vi "test - Enum.vi"(8 "error in (no error)":errorcluster, 11 "TestCase in":refnum<class "testcase-Supported-Datatype.lvclass">) -> (0 "error out":errorcluster, 3 "TestCase out":refnum<class "testcase-Supported-Datatype.lvclass">)   [LabVIEW 2017, in "testcase-Supported-Datatype.lvclass"]
uses:
  testcase-Supported-Datatype.lvclass
  <vilib>/addons/_JKI Toolkits/VI Tester/TestCase.llb/TestCase.lvclass
  addons/API-String-Arugments-Support/API String Arguments Support.lvlib
  C:/Program Files (x86)/National Instruments/LabVIEW 2017/vi.lib/addons/_JKI Toolkits/VI Tester/TestCase.llb/TestCase.lvclass
panel:
  out "data 3":enum16{"1 - aaaa", "2 - bbbb", "555 - ccccc"}(ring)
  out "data 2":enum16{"1 - aaaa", "2 - bbbb", "555 - ccccc"}(ring)
  out "data":enum16{"aaaa", "bbbb", "ccccc"}(ring)
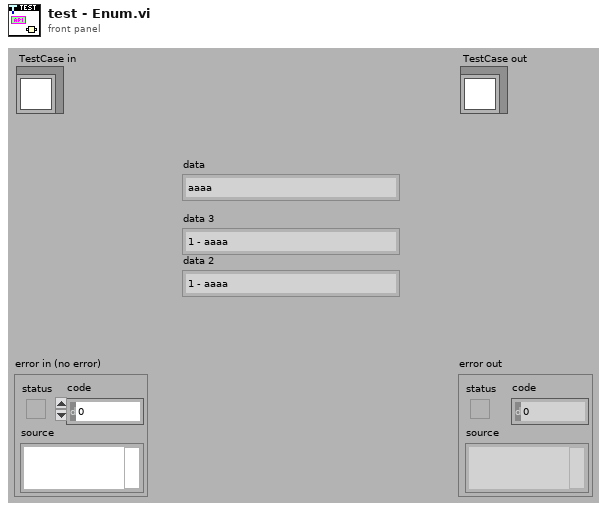
[diagram p1: front panel]
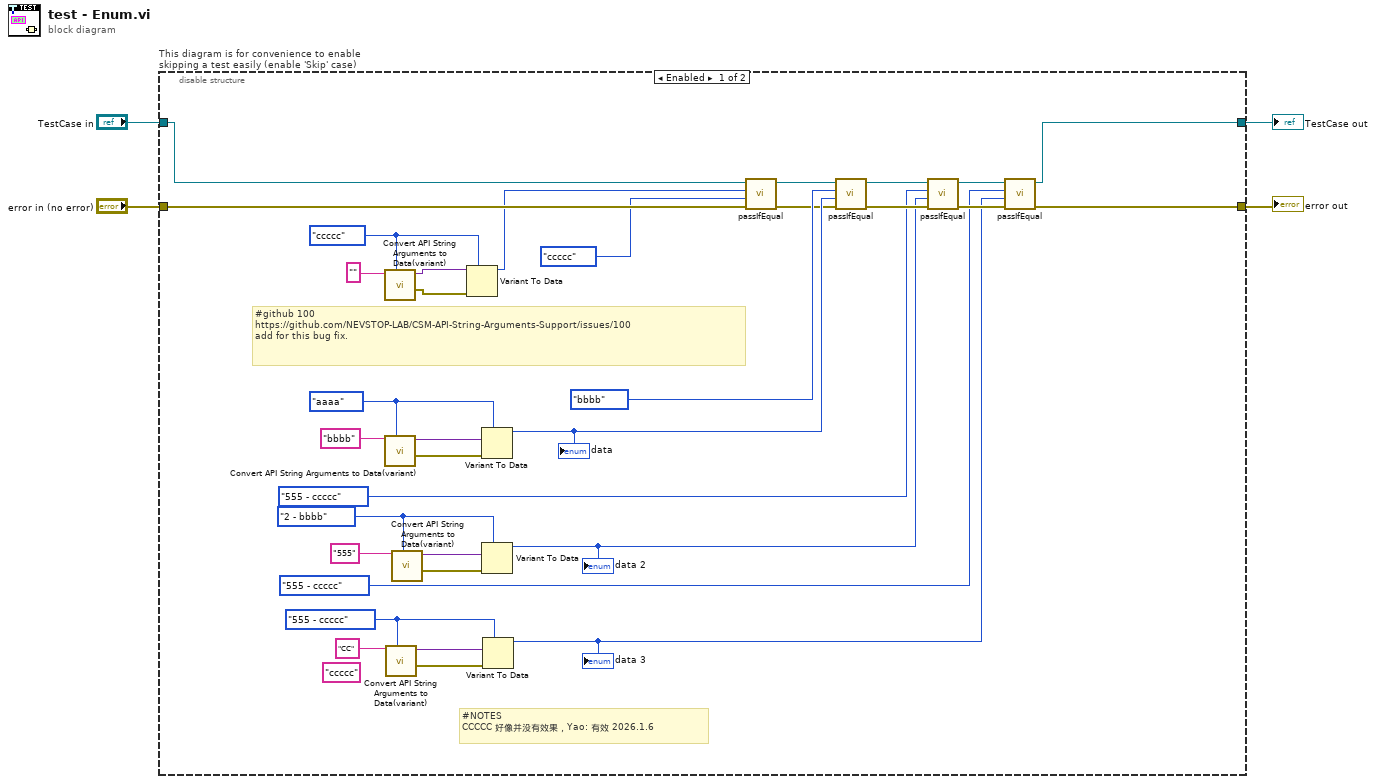
[diagram p0: block diagram]
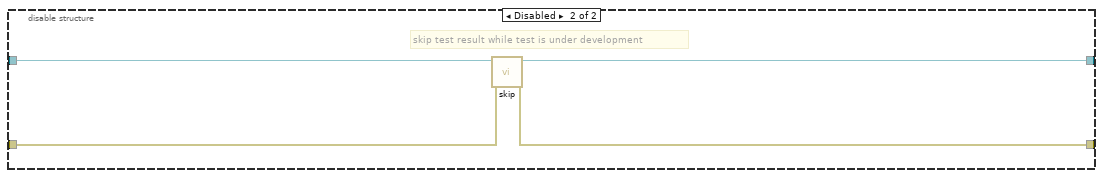
[diagram p2: hidden frame]
diagram:
  n1 = disable-structure "This diagram is for convenience to enable skipping a test easily (enable 'Skip' case)" shown="Enabled" {
    disable-tunnel: "TestCase in" -> [w14 w42]
    disable-tunnel: [w18 w40] -> w1
    disable-tunnel: [w17 w41] -> w3
    disable-tunnel: "error in (no error)" -> [w13 w39]
    frame Enabled {
      (unwired) "ccccc" ("String")
      w7 = enum16{"aaaa", "bbbb", "ccccc"}."ccccc" ("Data 5")
      w21 = enum16{"1 - aaaa", "2 - bbbb", "555 - ccccc"}."555 - ccccc" ("Data 6")
      w29 = enum16{"1 - aaaa", "2 - bbbb", "555 - ccccc"}."2 - bbbb" ("Data 6")
      w35 = enum16{"aaaa", "bbbb", "ccccc"}."aaaa" ("Data 5")
      # "#github 100\nhttps://github.com/NEVSTOP-LAB/CSM-API-String-Arguments-Support/issues/100\nadd for this bug fix."
      # "#NOTES\nCCCCC 好像并没有效果，Yao: 有效 2026.1.6"
      n2 = call "Convert API String Arguments to Data(variant).vi"("Type"=w7, "String"="") -> ("error"=w8:errorcluster, "Data"=w9:variant)  [unwired: 8 in]
      n3 = call "Convert API String Arguments to Data(variant).vi"("Type"=w35, "String"="bbbb") -> ("error"=w38:errorcluster, "Data"=w37:variant)  [unwired: 8 in]
      n4 = call "Convert API String Arguments to Data(variant).vi"("Type"=w21, "String"="CC") -> ("error"=w22:errorcluster, "Data"=w23:variant)  [unwired: 8 in]
      n5 = call "Convert API String Arguments to Data(variant).vi"("Type"=w29, "String"="555") -> ("error"=w30:errorcluster, "Data"=w31:variant)  [unwired: 8 in]
      n6 = Variant To Data(error in=w8, type=w7, Variant=w9) -> (data=w6:enum16{"aaaa", "bbbb", "ccccc"})  [unwired: 1 out]
      n7 = Variant To Data(error in=w38, type=w35, Variant=w37) -> (data=w33:enum16{"aaaa", "bbbb", "ccccc"})  [unwired: 1 out]
      "data" <- w33
      n8 = Variant To Data(error in=w30, type=w29, Variant=w31) -> (data=w25:enum16{"1 - aaaa", "2 - bbbb", "555 - ccccc"})  [unwired: 1 out]
      "data 2" <- w25
      n9 = Variant To Data(error in=w22, type=w21, Variant=w23) -> (data=w15:enum16{"1 - aaaa", "2 - bbbb", "555 - ccccc"})  [unwired: 1 out]
      "data 3" <- w15
      n10 = call-dynamic "passIfEqual.vi"("error in (no error)"=w13, "y"=enum16{"aaaa", "bbbb", "ccccc"}."ccccc" ("Data 5"), "x"=w6, "TestCase in"=w14) -> ("error out"=w12:errorcluster, "TestCase out"=w11:refnum<class "testcase-Supported-Datatype.lvclass">)  [unwired: 6 in]
      n11 = call-dynamic "passIfEqual.vi"("error in (no error)"=w12, "y"=w33, "x"=enum16{"aaaa", "bbbb", "ccccc"}."bbbb" ("Data 5"), "TestCase in"=w11) -> ("error out"=w28:errorcluster, "TestCase out"=w27:refnum<class "testcase-Supported-Datatype.lvclass">)  [unwired: 6 in]
      n12 = call-dynamic "passIfEqual.vi"("error in (no error)"=w28, "y"=w25, "x"=enum16{"1 - aaaa", "2 - bbbb", "555 - ccccc"}."555 - ccccc" ("Data 6"), "TestCase in"=w27) -> ("error out"=w19:errorcluster, "TestCase out"=w20:refnum<class "testcase-Supported-Datatype.lvclass">)  [unwired: 6 in]
      n13 = call-dynamic "passIfEqual.vi"("error in (no error)"=w19, "y"=w15, "x"=enum16{"1 - aaaa", "2 - bbbb", "555 - ccccc"}."555 - ccccc" ("Data 6"), "TestCase in"=w20) -> ("error out"=w17:errorcluster, "TestCase out"=w18:refnum<class "testcase-Supported-Datatype.lvclass">)  [unwired: 6 in]
    }
    frame Disabled {
      # "skip test result while test is under development"
      n14 = call <vilib>:"skip.vi"("error in (no error)"=w39, "TestCase in"=w42) -> ("error out"=w41:errorcluster, "TestCase out"=w40:refnum<class "testcase-Supported-Datatype.lvclass">)  [unwired: 8 in]
    }
  }
  "error out" <- w3
  "TestCase out" <- w1
